vi "DBC-GET-IDX-BY-TAG.vi"(8 "error in (no error)":errorcluster, 9 "tag":string, 11 "dbc in":refnum<class "dbc.lvclass">) -> (0 "error out":errorcluster, 1 "Numeric":i32, 3 "dbc out":refnum<class "dbc.lvclass">)   [LabVIEW 2015, in "dbc.lvclass"]
uses:
  dbc.lvclass
  dbc.lvclass/dbc.ctl
  read-tree-ref.vi
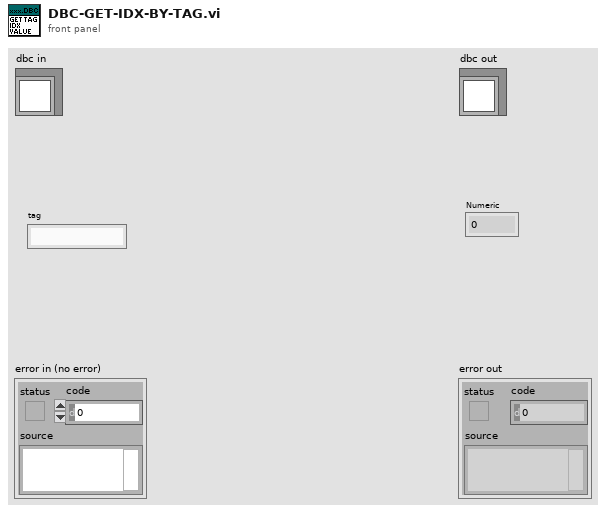
[diagram p1: front panel]
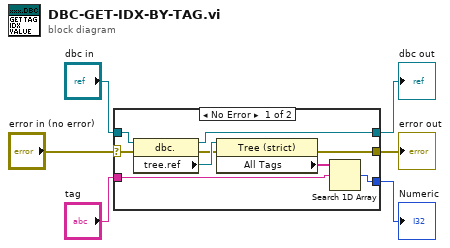
[diagram p0: block diagram]
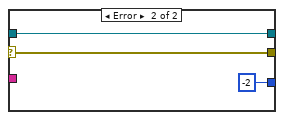
[diagram p2: hidden frame]
diagram:
  n1 = case shown="No Error" "error in (no error)" {
    selector: "error in (no error)" -> [w8 w18]
    tunnel: [w7 w18] -> w5
    tunnel: [w14 w17] -> w3
    tunnel: "dbc in" -> [w15 w17]
    tunnel: "tag" -> [w11 _]
    tunnel: [w10 -2] -> w1
    frame No Error {
      n2 = property class="dbc."(reference=w15, error in=w8) -> (reference out=w14:refnum<class "dbc.lvclass">, error out=w9:errorcluster, "tree.ref"=w13:refnum<vi>)
      n3 = property class="Tree (strict)"(reference=w13, error in=w9) -> (error out=w7:errorcluster, "All Tags"=w12:string[])  [unwired: 1 out]
      n4 = Search 1D Array(1D array=w12, element=w11) -> (index of element=w10:i32)  [unwired: 1 in]
    }
    frame Error {
    }
  }
  "error out" <- w5
  "dbc out" <- w3
  "Numeric" <- w1
